vi "Build_m_script.vi"(4 "oPENpdf":bool, 10 "String in":string, 11 "path to JPEG file":path) -> (3 "String out":string)   [LabVIEW 2023]
doc: "Genere le fichier pdf"
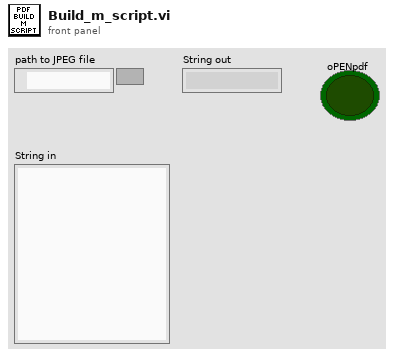
[diagram p1: front panel]
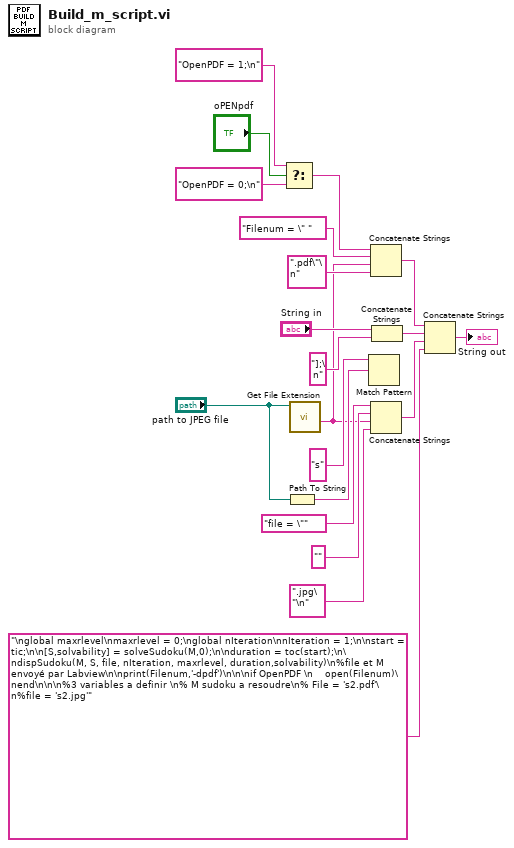
[diagram p0: block diagram]
diagram:
  n1 = Select(t="OpenPDF = 1;\n" ("string"), s="oPENpdf", f="OpenPDF = 0;\n" ("string")) -> (s? t:f=w4:string)
  n2 = Path To String(path="path to JPEG file") -> (string=w11:string)
  n3 = call <vilib>:"Get File Extension.vi"("file"="path to JPEG file") -> ("filename without extension"=w5:string)  [unwired: 6 in, 4 out]
  n4 = Match Pattern(string="s", regular expression=w11) -> ()  [unwired: 1 in, 4 out]
  n5 = Concatenate Strings(w4, "Filenum = \" " ("string"), w5, ".pdf\"\n" ("string")) -> (w14:string)
  n6 = Concatenate Strings("file = \"" ("string"), "" ("string"), w5, ".jpg\"\n" ("string")) -> (w19:string)
  n7 = Concatenate Strings("String in", "];\n" ("string")) -> (w9:string)
  n8 = Concatenate Strings(w14, w9, w19, "\nglobal maxrlevel\nmaxrlevel = 0;\nglobal nIteration\nnIteration = 1;\n\nstart = tic;\n\n[S,solvability] = solveSudoku(M,0);\n\nduration = toc(start);\n\ndispSudoku(M, S, file, nIteration, maxrlevel, duration,solvability)\n%file et M envoyé par Labview\n\nprint(Filenum,'-dpdf')\n\n\nif OpenPDF \n    open(Filenum)\nend\n\n\n%3 variables a definir \n% M sudoku a resoudre\n% File = 's2.pdf'\n%file = 's2.jpg'" ("string")) -> (→"String out":string)
